vi "ziExample-Module-Impedance.vi"() -> ()   [LabVIEW 2009]
doc: "Control a Zurich instrument device via the LabOne Labview API. \nRequirements: Zurich Instruments MFLI+IA/ MFIA\nThis example shows how to use retrieve impedance data and utilize the sweeper.\n\n© Zurich Instruments AG, www.zhinst.com"
uses:
  <instrlib>/Zurich Instruments LabOne/Public/Modules/ziTypeModSweeperImpedanceWave.ctl
  <instrlib>/Zurich Instruments LabOne/Public/Modules/ziTypeModEnum.ctl
  <instrlib>/Zurich Instruments LabOne/Public/Configure/ziSetValueDoubleArray.vi
  <instrlib>/Zurich Instruments LabOne/Public/Modules/ziModSetValueDoubleArray.vi
  <instrlib>/Zurich Instruments LabOne/Public/Modules/ziModSetValueBinaryArray.vi
  <instrlib>/Zurich Instruments LabOne/Public/Modules/ziModGetSweeperData.vi
  <instrlib>/Zurich Instruments LabOne/Public/Data/ziGetEventImpSample.vi
  <instrlib>/Zurich Instruments LabOne/Public/Configure/ziGetValueDouble.vi
  <instrlib>/Zurich Instruments LabOne/Public/Configure/ziSetValueDouble.vi
  <instrlib>/Zurich Instruments LabOne/Zurich Instruments LabOne.lvlib
  <vilib>/gmath/NI_Gmath.lvlib
panel:
  out "Frequency":dbl
  in  "auto/inputrange":bool caption="Auto"
  in  "voltage/range":dbl=1.0 caption="Range Voltage"
  in  "current/range":dbl=0.001 caption="Range Current"
  in  "output/amplitude":dbl=0.1 caption="Test Signal (V)"
  in  "auto/output":bool caption="Auto"
  in  "model":u16(ring)=1 caption="Model" items=["Rp || Cp", "Rs + Cs", "Rs + Ls", "G B", "D Cs", "Q Cs", "D Ls", "Q Ls", "Rp || Lp", "D Cp"]
  out "?":dbl(graph)
  out "?":dbl(graph)
  in  "Sweep":bool
  in  "Step":dbl=100.0
  in  "stopfreq":dbl=100000.0 caption="Stop Freq"
  in  "startfreq":dbl=1000.0 caption="Start Freq"
  out "Flags":bool[][](array[boolean])
  out "ImpedanceSweeperData":T1 {"bandwidthMode" format="%f"; "flags" format="%f"; "sampleFormat" format="%f"; "sweepMode" format="%f"; "sampleCount" format="%f"; "timestamp" format="%f"}
  in  "stop":bool
  out "IA Parameter 2":dbl
  out "IA Parameter 1":dbl format="%#_6p"
  out "Error Out":errorcluster
  in  "Address":string="DEV"
  out "Selected Device":string
  in  "subscribepath":string="imps/0/sample" caption="Subscribe Path"
  out "Param1":cluster{"grid":dbl[], "r_avg":dbl[]}(graph)
  out "Param 0":cluster{"grid":dbl[], "r_avg":dbl[]}(graph)
  # "ziExample-IMPModul.vi\nRequirements: MFLI + IA / MFIA\nsee block diagram for VI description"
  # "Tested Devices:\n\n- MFLI"
  # "VALID_INTERNAL\nVALID_USER\nAUTORANGE_GATING\n\nOVERFLOW_VOLTAGE\nOVERFLOW_CURRENT\nUNDERFLOW_VOLTAGE\nUNDERFLOW_CURRENT\nFREQ_EXACT\nFREQ_INTERPOLATION\nFREQ_EXTRAPOLATION\n\nSUPPRESSION_PARAM0\nSUPPRESSION_PARAM1\nFREQLIMIT_RANGE_VOLTAGE\nFREQLIMIT_RANGE_Current\nSTRONGCOMPENSATION_PARAM0\nSTRONGCOMPENSATION_PARAM1\n\n\nBWC_BIT0\nBWC_BIT1\nBWC_BIT2\nBWC_BIT3\nOPEN_DETECTION"
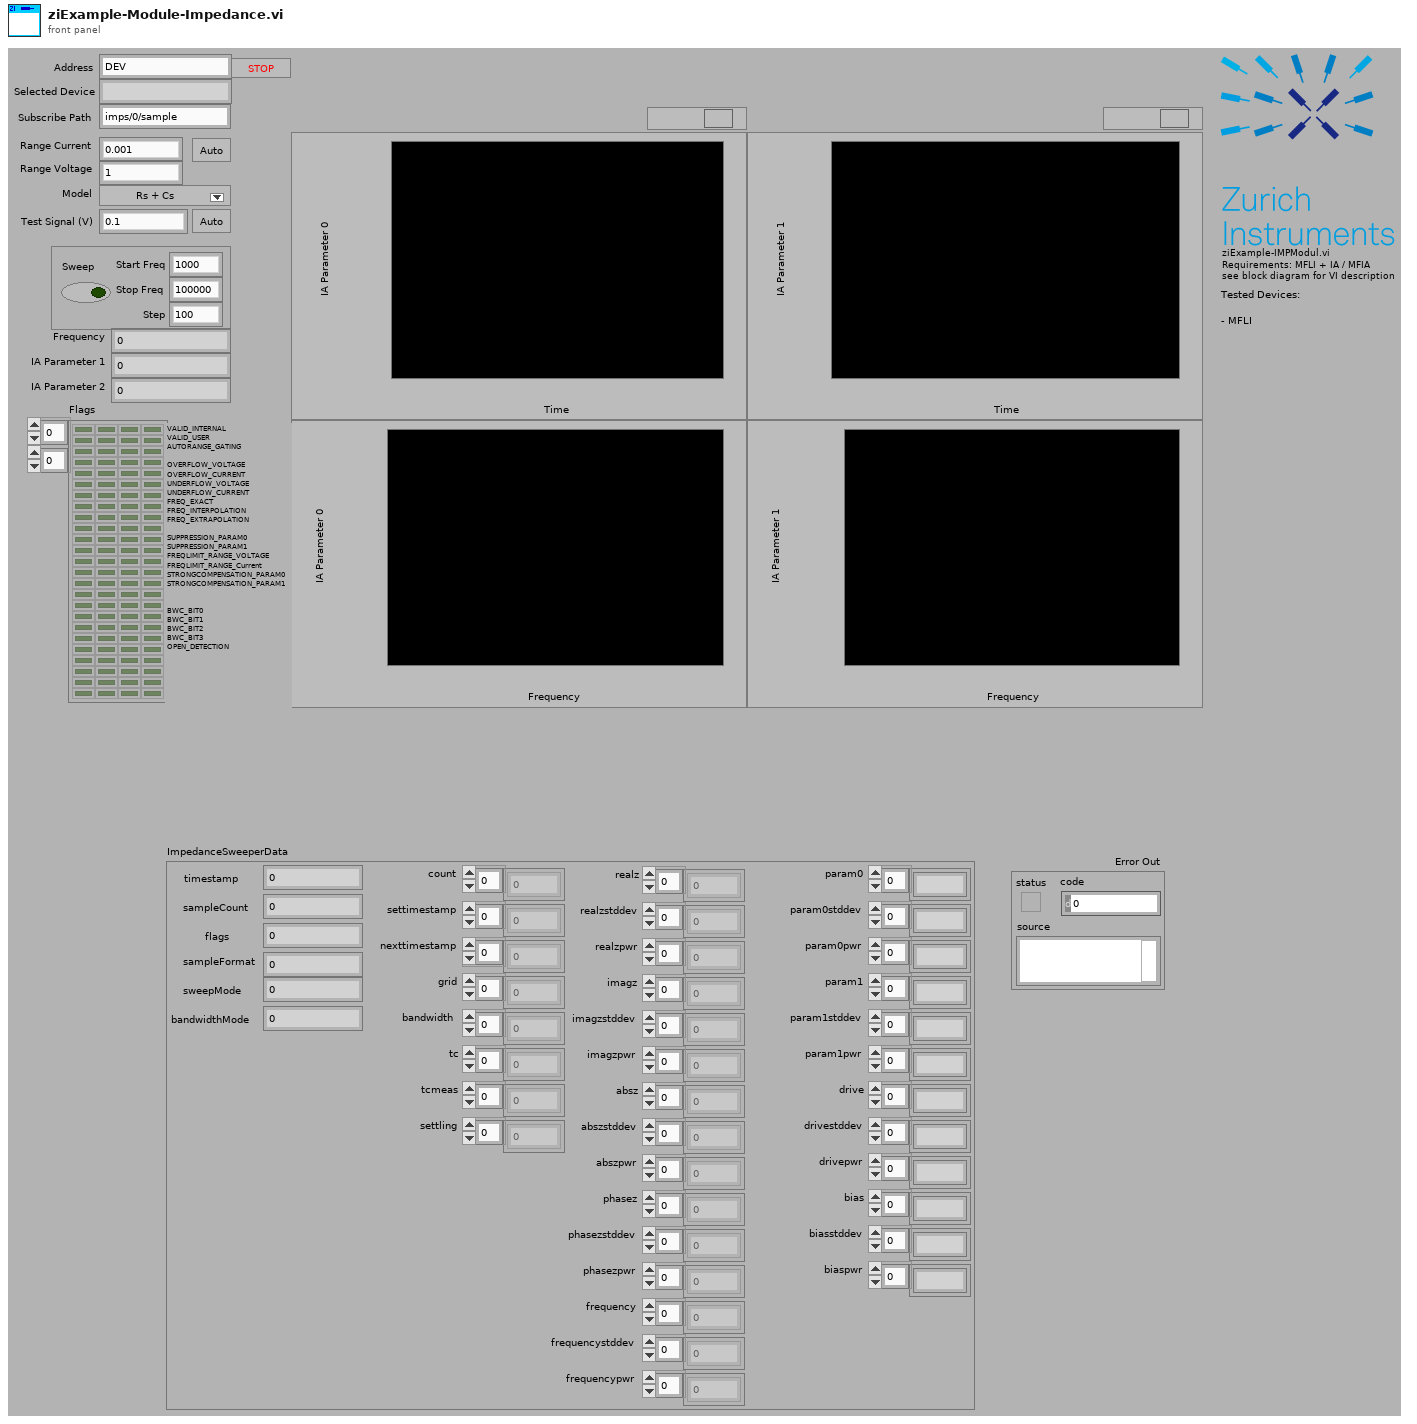
[diagram p1: front panel]
types:
  T1 = typedef "Zurich Instruments LabOne.lvlib/ziTypeModSweeperImpedanceWave.ctl" = cluster{"timestamp":u64, "sampleCount":u64, "flags":u8, "sampleFormat":u8, "sweepMode":u8, "bandwidthMode":u8, "count":u64[], "settimestamp":u64[], "nexttimestamp":u64[], "grid":dbl[], "bandwidth":dbl[], "tc":dbl[], "tcmeas":dbl[], "settling":dbl[], "realz":dbl[], "realzstddev":dbl[], "realzpwr":dbl[], "imagz":dbl[], "imagzstddev":dbl[], "imagzpwr":dbl[], "absz":dbl[], "abszstddev":dbl[], "abszpwr":dbl[], "phasez":dbl[], "phasezstddev":dbl[], "phasezpwr":dbl[], "frequency":dbl[], "frequencystddev":dbl[], "frequencypwr":dbl[], "param0":dbl[], "param0stddev":dbl[], "param0pwr":dbl[], "param1":dbl[], "param1stddev":dbl[], "param1pwr":dbl[], "drive":dbl[], "drivestddev":dbl[], "drivepwr":dbl[], "bias":dbl[], "biasstddev":dbl[], "biaspwr":dbl[]}
  T2 = typedef "Zurich Instruments LabOne.lvlib/ziTypeModEnum.ctl" = u16
  T3 = typedef "Zurich Instruments LabOne.lvlib/ziTypeHandle.ctl" = cluster{"handleValid":bool, "Conn":u64, "Path Prefix":string, "Handle":u64, "Connected":bool, "Clockbase(s)":dbl}
  T4 = typedef "Zurich Instruments LabOne.lvlib/ziTypeModHandle.ctl" = cluster{"handleValid":bool, "Conn":u64, "ModHandle":u64, "moduleID":string, "Path Prefix":string}
  T5 = typedef "Zurich Instruments LabOne.lvlib/ziTypeModResults.ctl" = cluster{"PathArray":string[], "ValueType":T6, "NoOfResults":u64, "ziGenericHeader":T7[]}
  T6 = typedef "Zurich Instruments LabOne.lvlib/ziTypePollType.ctl" = enum16{"NONE", "DOUBLE_DATA", "INTEGER_DATA", "DEMOD_SAMPLE", "SCOPE_WAVE_HF2", "AUXIN_SAMPLE", "DIO_SAMPLE", "BYTE_ARRAY", "PWA_WAVE", "9", "10", "11", "12", "13", "14", "15", "TREE_CHANGE_DEPRI", "17", "ERROR", "19", "20", "21", "22", "23", "24", "25", "26", "27", "28", "29", "30", "31", "DOUBLE_DATA_TS", "INTEGER_DATA_TS", "34", "SCOPE_WAVE", "SCOPE_WAVE_EX", "37", "BYTE_ARRAY_TS", "39", "40", "41", "42", "43", "44", "45", "CNT_DATA", "47", "TREE_CHANGE", "49", "50", "51", "52", "53", "54", "55", "56", "57", "58", "59", "60", "61", "62", "63", "SWEEPER_DATA", "SPECTRUM_DATA", "ADVISOR_DATA", "VECTOR_DATA", "IMP_DATA"}
  T7 = typedef "Zurich Instruments LabOne.lvlib/ziTypeModGenericHeader.ctl" = cluster{"HeaderType":enum8{"HEADER_TYPE_NONE", "HEADER_TYPE_SWTRIGGER", "HEADER_TYPE_SWEEPER"}, "SampleFormat":u8, "SystemTime":timestamp, "CreatedTimeStamp":u64, "ChangedTimeStamp":u64, "Flags":u32, "ChunkSizeBytes":u64, "Name":string, "Status":u32, "GroupIndex":u32, "Color":u32, "ActiveRow":u32, "TriggerNumber":u64, "GridRows":u32, "GridCols":u32, "GridMode":u32, "GridOperation":u32, "GridDirection":u32, "GridRepetitions":u32, "GridColDelta":dbl, "GridColOffset":dbl, "GridRowDelta":dbl, "GridRowOffset":dbl, "Bandwidth":dbl, "Center":dbl, "Nenbw":dbl}
  T8 = typedef "Zurich Instruments LabOne.lvlib/ziTypeImpedanceSample.ctl" = cluster{"Timestamps (ticks)":u64[], "Z (Ohm)":cdb[], "Freq (Hz)":dbl[], "Osc Phase (deg)":dbl[], "Flags":u32[], "Trigger":u32[], "Param0":dbl[], "Param1":dbl[], "Drive":dbl[], "Bias":dbl[]}
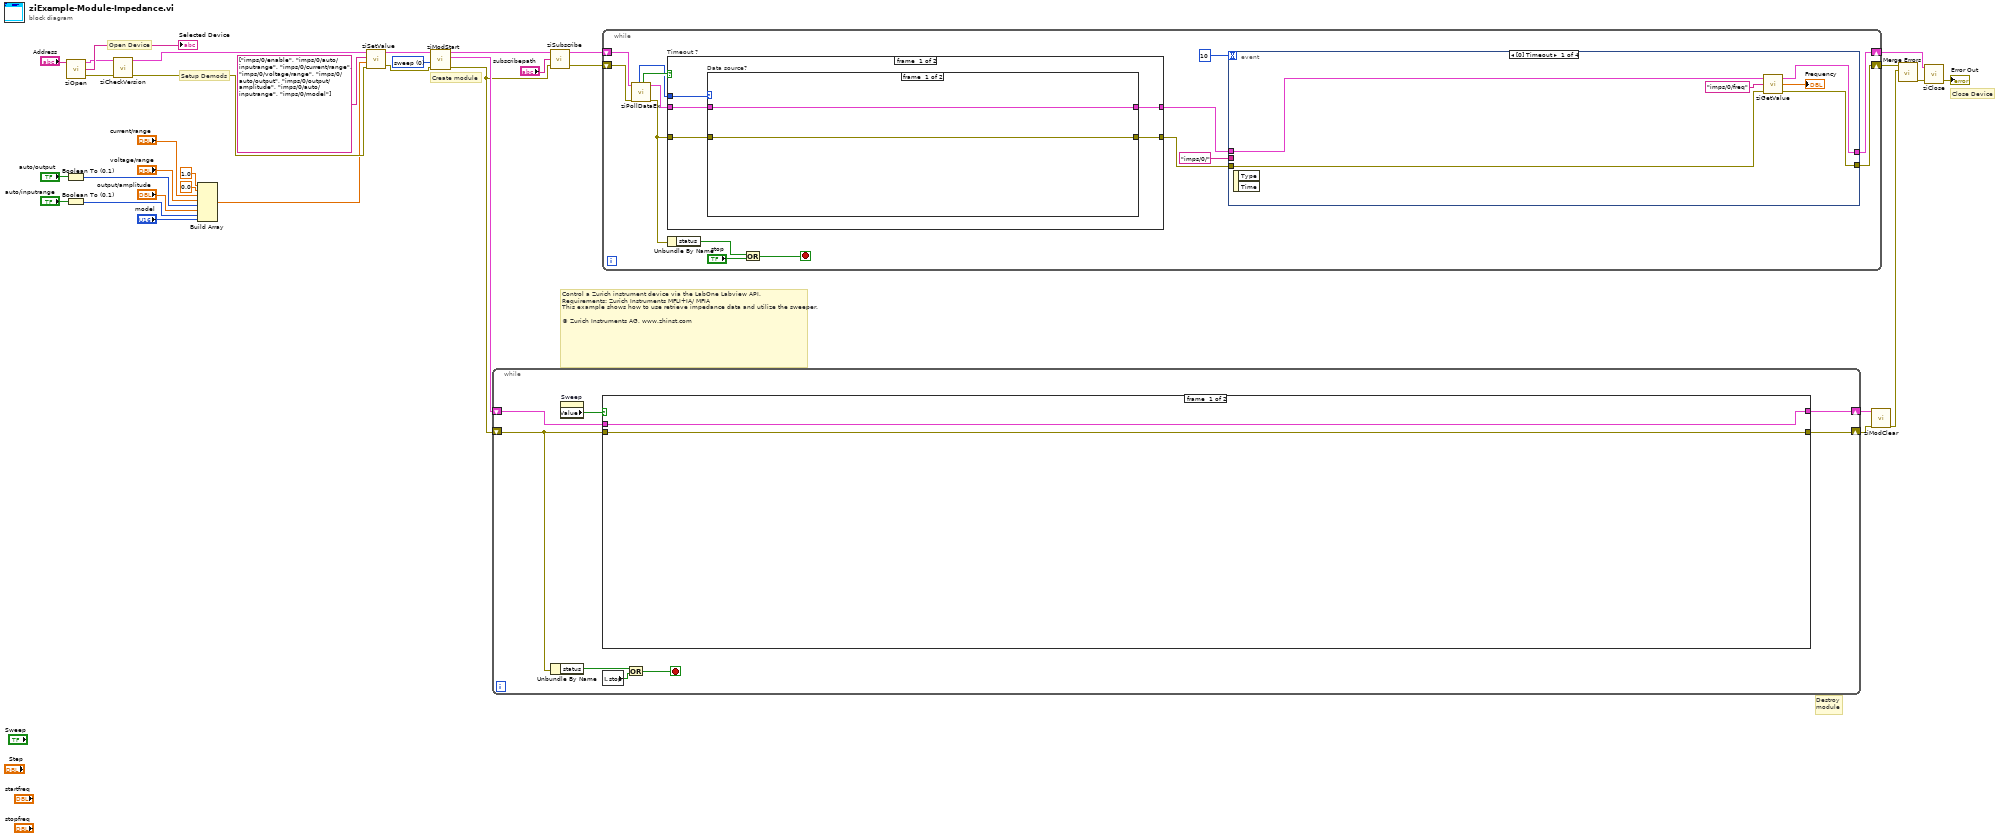
[diagram p0: block diagram]
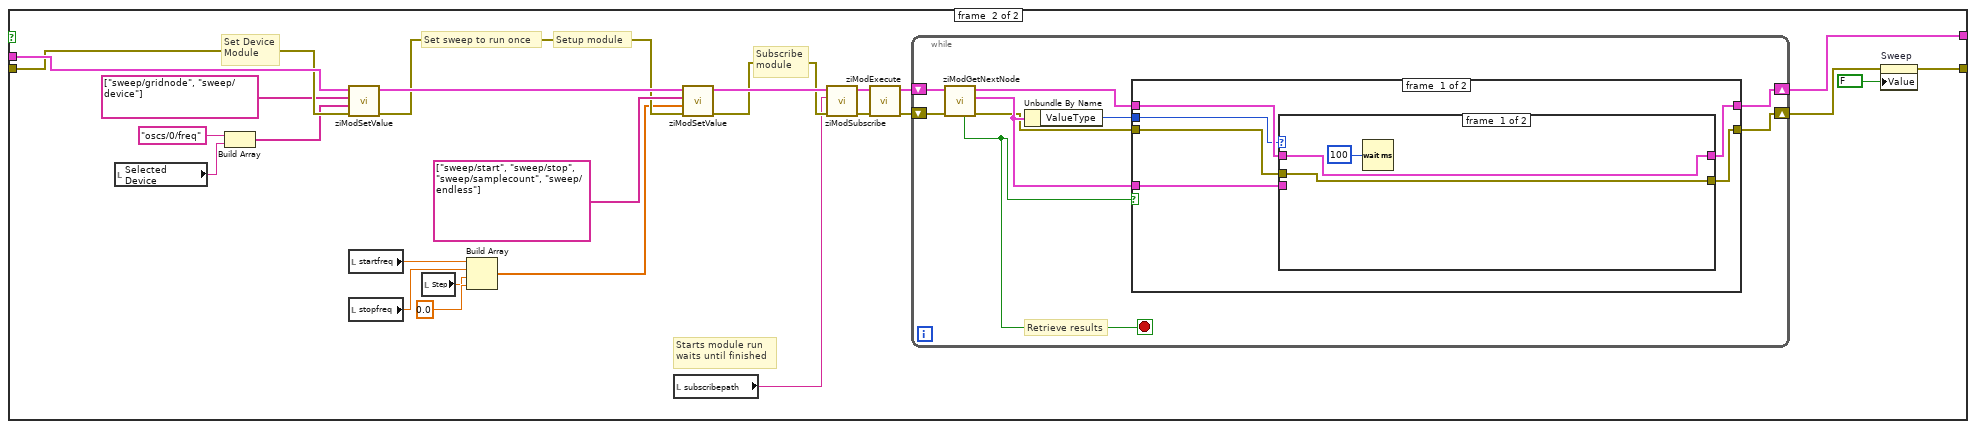
[diagram p2: hidden frame]
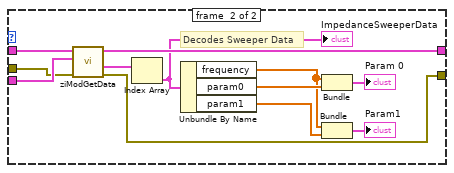
[diagram p3: hidden frame]
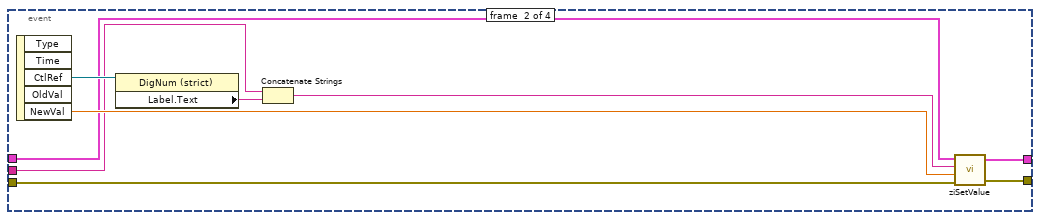
[diagram p5: hidden frame]
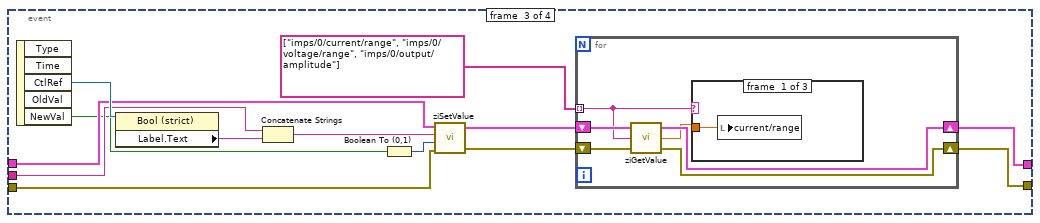
[diagram p6: hidden frame]
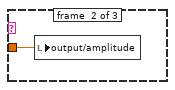
[diagram p7: hidden frame]
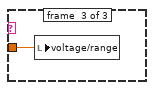
[diagram p8: hidden frame]
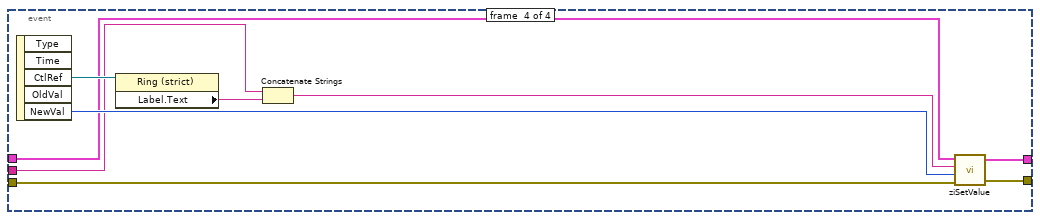
[diagram p9: hidden frame]
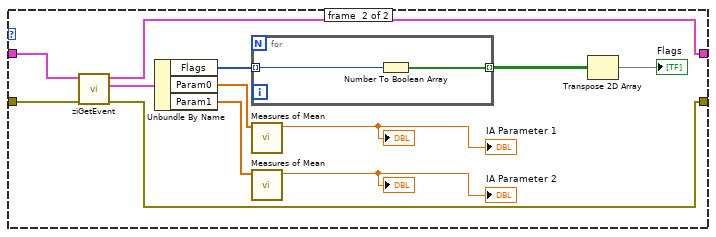
[diagram p10: hidden frame]
diagram:
  w15 = T2 0 items=["sweep", "scopeModule", "dataAcquisitionModule", "pidAdvisor", "awgModule", "impedanceModule", "multiDeviceSyncModule", "zoomFFT", "trigger", "deviceSettings", "record"] ("module Id")
  # "Destroy\nmodule"
  # "Control a Zurich instrument device via the LabOne Labview API. \nRequirements: Zurich Instruments MFLI+IA/ MFIA\nThis example shows how to use retrieve impedance data and utilize the sweeper.\n\n© Zurich Instruments AG, www.zhinst.com"
  # "Setup Demods"
  # "Create module"
  # "Close Device"
  # "Open Device"
  n1 = Boolean To (0,1)(Boolean="auto/output") -> (0, 1=w7:i16)
  n2 = Boolean To (0,1)(Boolean="auto/inputrange") -> (0, 1=w8:i16)
  n3 = call <instrlib>:"ziOpen.vi"("Address"="Address") -> ("Error Out"=w18:errorcluster, "Selected Device"=→"Selected Device":string, "HandleOut"=w19:T3)  [unwired: 1 in, 2 out]
  n4 = call <instrlib>:"ziCheckVersion.vi"("Handle In"=w19, "Error In"=w18) -> ("Handle Out"=w16:T3, "Error Out"=w17:errorcluster)  [unwired: 11 in, 1 out]
  n5 = Build Array(1.0 ("element"), 0.0 ("element"), "current/range", "voltage/range", w7, "output/amplitude", w8, "model") -> (w3:dbl[])
  n6 = call-poly <instrlib>:"ziSetValue.vi"("Error In"=w17, "Values"=w3, "Paths"=string[] ["imps/0/enable", "imps/0/auto/inputrange", "imps/0/current/range", "imps/0/voltage/range", "imps/0/auto/output", "imps/0/output/amplitude", "imps/0/auto/inputrange", "imps/0/model"], "Handle In"=w16) -> ("Error Out"=w20:errorcluster, "Handle Out"=w21:T3)  [unwired: 1 in]
  n7 = call <instrlib>:"ziModStart.vi"("Error In"=w20, "module Id"=w15, "Handle In"=w21) -> ("Error Out"=w26:errorcluster, "ModHandle Out"=w33:T4, "Handle Out"=w29:T3)  [unwired: 6 in]
  n8 = while {
    shift-right: [w40] -> w31
    shift-left: w33 -> [w42]
    shift-right: [w41] -> w32
    shift-left: w26 -> [w38]
    stop <- w35 stop-if-true
    n9 = Unbundle By Name(w38) -> ("status"=w36:bool)
    n10 = property on="Sweep" class="Bool (strict)"() -> ("Value"=w39:bool)  [unwired: 2 in, 2 out]
    n11 = case shown="False" w39 {
      tunnel: w42 -> [w44 w69]
      tunnel: [w43 w68] -> w41
      tunnel: [w44 w67] -> w40
      tunnel: w38 -> [w43 w66]
      frame #0 {
      }
      frame #1 {
        # "Set Device\nModule"
        # "Starts module run\nwaits until finished"
        # "Set sweep to run once"
        # "Subscribe\nmodule"
        # "Setup module"
        n12 = local read "Selected Device"() -> (w53:string)
        n13 = Build Array("oscs/0/freq", w53) -> (w51:string[])
        n14 = call-poly <instrlib>:"ziModSetValue.vi"("Error In"=w66, "Values"=w51, "Paths"=string[] ["sweep/gridnode", "sweep/device"], "ModHandle In"=w69) -> ("Error Out"=w59:errorcluster, "ModHandle Out"=w62:T4)  [unwired: 6 in]
        n15 = local read "startfreq"() -> (w47:dbl)
        n16 = local read "stopfreq"() -> (w46:dbl)
        n17 = local read "Step"() -> (w45:dbl)
        n18 = Build Array(w47, w46, w45, 0.0 ("Value")) -> (w54:dbl[])
        n19 = local read "subscribepath"() -> (w58:string)
        n20 = call-poly <instrlib>:"ziModSetValue.vi"("Error In"=w59, "Values"=w54, "Paths"=string[] ["sweep/start", "sweep/stop", "sweep/samplecount", "sweep/endless"], "ModHandle In"=w62) -> ("Error Out"=w60:errorcluster, "ModHandle Out"=w61:T4)  [unwired: 6 in]
        n21 = call <instrlib>:"ziModSubscribe.vi"("Error In"=w60, "Path"=w58, "ModHandle In"=w61) -> ("Error Out"=w55:errorcluster, "ModHandle Out"=w56:T4)  [unwired: 6 in]
        n22 = call <instrlib>:"ziModExecute.vi"("Error In"=w55, "ziModHandle In"=w56) -> ("Error Out"=w64:errorcluster, "ziModHandle Out"=w65:T4)  [unwired: 6 in, 1 out]
        n23 = while {
          shift-right: [w75] -> w67
          shift-left: w65 -> [w77]
          shift-right: [w74] -> w49
          shift-left: w64 -> [w78]
          stop <- w70 stop-if-true
          # "Retrieve results"
          n24 = call <instrlib>:"ziModGetNextNode.vi"("Error In"=w78, "ModHandle In"=w77) -> ("Error Out"=w71:errorcluster, "ModResults"=w73:T5, "ModHandle Out"=w76:T4, "NoData"=w70:bool)  [unwired: 6 in]
          n25 = Unbundle By Name(w73) -> ("ValueType"=w72:T6)
          n26 = case shown="False" w70 {
            tunnel: w76 -> [w84 w100]
            tunnel: [w83 w100] -> w75
            tunnel: [w82 w101] -> w74
            tunnel: w71 -> [w81 w101]
            tunnel: w73 -> [w80 _]
            tunnel: w72 -> [w79 _]
            frame #0 {
              n27 = case shown="\"SWEEPER_DATA\"" w79 {
                tunnel: w84 -> [w87 w98]
                tunnel: w80 -> [_ w99]
                tunnel: w81 -> [w86 w97]
                tunnel: [w86 w96] -> w82
                tunnel: [w87 w95] -> w83
                frame #0 {
                  n28 = Wait (ms)(milliseconds to wait=u32 100) -> ()  [unwired: 1 out]
                }
                frame #1 {
                  # "Decodes Sweeper Data"
                  n29 = call-poly <instrlib>:"ziModGetData.vi"("Error In"=w97, "ModResults"=w99, "ModHandle In"=w98) -> ("Error Out"=w96:errorcluster, "SweeperImpedanceWaveArray"=w89:T1[], "ModHandle Out"=w95:T4)  [unwired: 4 in, 2 out]
                  n30 = Index Array(array=w89) -> (element=w88:T1)  [unwired: 1 in]
                  "ImpedanceSweeperData" <- w88
                  n31 = Unbundle By Name(w88) -> ("frequency"=w90:dbl[], "param0"=w94:dbl[], "param1"=w91:dbl[])
                  n32 = Bundle("frequency"=w90, "param0"=w94) -> (→"Param 0":cluster{"frequency":dbl[], "param0":dbl[]})  [unwired: 1 in]
                  n33 = Bundle("frequency"=w90, "param1"=w91) -> (→"Param1":cluster{"frequency":dbl[], "param1":dbl[]})  [unwired: 1 in]
                }
              }
            }
            frame #1 {
            }
          }
        }
        n34 = property on="Sweep" class="Bool (strict)"(error in=w49, "Value"=FALSE ("Sweep")) -> (error out=w68:errorcluster)  [unwired: 1 in, 1 out]
      }
    }
    n35 = local read "stop"() -> (w37:bool)
    n36 = Or(x=w36, y=w37) -> (x .or. y?=w35:bool)
  }
  n37 = call <instrlib>:"ziSubscribe.vi"("error in"=w26, "Path ()"="subscribepath", "Handle In"=w29) -> ("error out"=w27:errorcluster, "Handle Out"=w28:T3)  [unwired: 1 in]
  n38 = while {
    shift-right: [w105] -> w24
    shift-left: w27 -> [w108]
    shift-right: [w106] -> w30
    shift-left: w28 -> [w109]
    stop <- w110 stop-if-true
    n39 = call <instrlib>:"ziPollDataEx.vi"("error in"=w108, "Handle In"=w109) -> ("error out"=w113:errorcluster, "Handle Out"=w115:T3, "Timed Out"=w116:bool, "ziValueType"=w114:T6)  [unwired: 2 in, 4 out]
    n40 = case "Timeout ?" shown="False" w116 {
      tunnel: w115 -> [w167 w185]
      tunnel: [w166 w185] -> w107
      tunnel: w113 -> [w165 w184]
      tunnel: [w163 w184] -> w104
      tunnel: w114 -> [w164 _]
      frame #0 {
        n41 = case "Data source?" shown="\"IMP_DATA\"" w164 {
          tunnel: w167 -> [w169 w181]
          tunnel: [w169 w177] -> w166
          tunnel: w165 -> [w168 w179]
          tunnel: [w168 w178] -> w163
          frame #0 {
          }
          frame #1 {
            n42 = call-poly <instrlib>:"ziGetEvent.vi"("Error In"=w179, "Handle In"=w181) -> ("Error Out"=w178:errorcluster, "Imp Sample Out"=w180:T8, "Handle Out"=w177:T3)  [unwired: 7 in]
            n43 = Unbundle By Name(w180) -> ("Flags"=w176:u32[], "Param0"=w173:dbl[], "Param1"=w172:dbl[])
            n44 = for {
              tunnel: w176 -> [w183] mode=indexing
              tunnel: [w182] -> w175 mode=indexing
              n45 = Number To Boolean Array(number=w183) -> (Boolean array=w182:bool[])
            }
            n46 = call <vilib>:"Measures of Mean.vi"("x array"=w173) -> ("mean value"=→"IA Parameter 1" →"?":dbl)  [unwired: 9 in, 1 out]
            n47 = call <vilib>:"Measures of Mean.vi"("x array"=w172) -> ("mean value"=→"IA Parameter 2" →"?":dbl)  [unwired: 9 in, 1 out]
            n48 = Transpose 2D Array(2D array=w175) -> (transposed array=→"Flags":bool[][])
          }
        }
      }
      frame #1 {
        # "Timeout, no action."
      }
    }
    n49 = Unbundle By Name(w113) -> ("status"=w111:bool)
    n50 = Or(x=w111, y="stop") -> (x .or. y?=w110:bool)
    n51 = event shown="[0] Timeout" {
      selector: _ -> [_ _ _ _]
      dyn-events: _ -> [_ _ _ _]
      timeout: 10 -> [_ _ _ _]
      tunnel: w107 -> [w120 w129 w142 w157]
      tunnel: [w119 w128 w134 w160] -> w106
      tunnel: [w118 w127 w133 w159] -> w105
      tunnel: w104 -> [w117 w126 w141 w158]
      tunnel: "imps/0/" -> [_ w125 w138 w154]
      event #0 {
        n52 = event-data() -> ()  [unwired: 1 in, 2 out]
        n53 = call-poly <instrlib>:"ziGetValue.vi"("error in"=w117, "Path"="imps/0/freq", "Handle in"=w120) -> ("error out"=w118:errorcluster, "Value"=→"Frequency":dbl, "Handle out"=w119:T3)
      }
      event #1 {
        n54 = event-data() -> ("CtlRef"=w131:refnum<vi>, "NewVal"=w130:dbl)  [unwired: 1 in, 3 out]
        n55 = property class="DigNum (strict)"(reference=w131) -> ("Label.Text"=w124:string)  [unwired: 1 in, 2 out]
        n56 = Concatenate Strings(w125, w124) -> (w123:string)
        n57 = call-poly <instrlib>:"ziSetValue.vi"("Error In"=w126, "Value"=w130, "Path"=w123, "Handle In"=w129) -> ("Error Out"=w127:errorcluster, "Handle Out"=w128:T3)  [unwired: 1 in]
      }
      event #2 {
        n58 = event-data() -> ("CtlRef"=w144:refnum<vi>, "NewVal"=w137:bool)  [unwired: 1 in, 3 out]
        n59 = property class="Bool (strict)"(reference=w144) -> ("Label.Text"=w139:string)  [unwired: 1 in, 2 out]
        n60 = Concatenate Strings(w138, w139) -> (w140:string)
        n61 = Boolean To (0,1)(Boolean=w137) -> (0, 1=w143:i16)
        n62 = call-poly <instrlib>:"ziSetValue.vi"("Error In"=w141, "Value"=w143, "Path"=w140, "Handle In"=w142) -> ("Error Out"=w135:errorcluster, "Handle Out"=w136:T3)  [unwired: 1 in]
        n63 = for {
          tunnel: string[] ["imps/0/current/range", "imps/0/voltage/range", "imps/0/output/amplitude"] -> [w148] mode=indexing
          shift-right: [w146] -> w133
          shift-left: w135 -> [w149]
          shift-right: [w147] -> w134
          shift-left: w136 -> [w150]
          n64 = call-poly <instrlib>:"ziGetValue.vi"("error in"=w149, "Path"=w148, "Handle in"=w150) -> ("error out"=w146:errorcluster, "Value"=w145:dbl, "Handle out"=w147:T3)
          n65 = case shown="\"imps/0/current/range\", Default" w148 {
            tunnel: w145 -> [w151 w152 w153]
            frame #0 {
              n66 = local write "current/range"(w151) -> ()
            }
            frame #1 {
              n67 = local write "output/amplitude"(w152) -> ()
            }
            frame #2 {
              n68 = local write "voltage/range"(w153) -> ()
            }
          }
        }
      }
      event #3 {
        n69 = event-data() -> ("CtlRef"=w162:refnum<vi>, "NewVal"=w161:u16)  [unwired: 1 in, 3 out]
        n70 = property class="Ring (strict)"(reference=w162) -> ("Label.Text"=w155:string)  [unwired: 1 in, 2 out]
        n71 = Concatenate Strings(w154, w155) -> (w156:string)
        n72 = call-poly <instrlib>:"ziSetValue.vi"("Error In"=w158, "Value"=w161, "Path"=w156, "Handle In"=w157) -> ("Error Out"=w159:errorcluster, "Handle Out"=w160:T3)  [unwired: 1 in]
      }
    }
  }
  n73 = call <instrlib>:"ziModClear.vi"("Error In"=w32, "ziModHandle In"=w31) -> ("Error Out"=w25:errorcluster)  [unwired: 7 in, 1 out]
  n74 = call <vilib>:"Merge Errors.vi"("error in 2 (no error)"=w25, "error in 1 (no error)"=w24) -> ("error out"=w23:errorcluster)  [unwired: 5 in]
  n75 = call <instrlib>:"ziClose.vi"("Error In"=w23, "Handle In"=w30) -> ("Error Out"=→"Error Out":errorcluster)  [unwired: 2 in, 1 out]
